vi "Pasco Turn.vi"(9 "Power":dbl, 10 "actual":dbl, 11 "desired":dbl) -> (1 "There":bool, 2 "right drive":dbl, 3 "left drive":dbl)   [LabVIEW 2012]
panel:
  out "turn right":bool
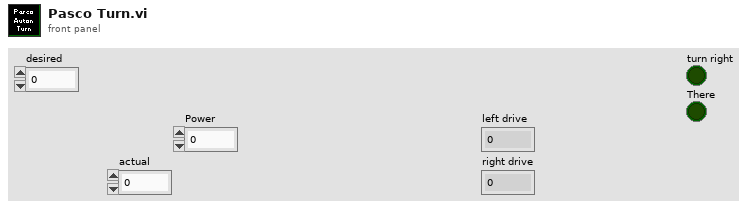
[diagram p1: front panel]
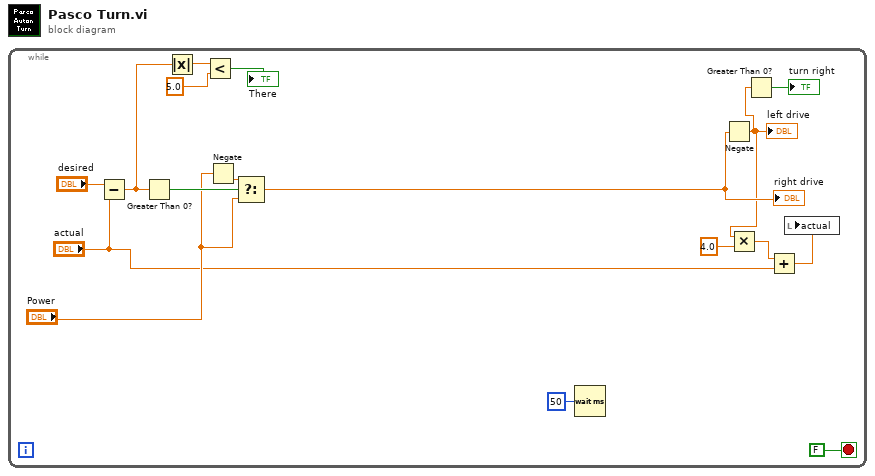
[diagram p0: block diagram]
diagram:
  n1 = while {
    stop <- FALSE stop-if-true
    n2 = Subtract(x="desired", y="actual") -> (x-y=w14:dbl)
    n3 = Greater Than 0?(x=w14) -> (x > 0?=w17:bool)
    n4 = Absolute Value(x=w14) -> (abs(x)=w12:dbl)
    n5 = Less?(x=w12, y=5.0) -> (x < y?=→"There":bool)
    n6 = Negate(x="Power") -> (-x=w16:dbl)
    n7 = Select(t=w16, s=w17, f="Power") -> (s? t:f=w15:dbl)
    "right drive" <- w15
    n8 = Wait (ms)(milliseconds to wait=u32 50) -> ()  [unwired: 1 out]
    n9 = Negate(x=w15) -> (-x=w3:dbl)
    "left drive" <- w3
    n10 = Multiply(x=w3, y=4.0) -> (x*y=w7:dbl)
    n11 = Greater Than 0?(x=w3) -> (x > 0?=→"turn right":bool)
    n12 = Add(x=w7, y="actual") -> (x+y=w10:dbl)
    n13 = local write "actual"(w10) -> ()
  }
